vi "sv_Uniquify Collection Name.vi"(0 "tdms file ref":refnum<k34>, 5 "collection name":string="FrequencyResponse", 7 "component names":string[](array[string])=["Magnitude", "Phase", "Coherence"], 11 "error in":errorcluster, 12 "separator":string="_") -> (4 "tdms file out":refnum<k34>, 6 "unique collection name":string, 8 "unique group names (collection_component)":string[](array[string]), 15 "error out":errorcluster)   [LabVIEW 2017]
uses:
  <vilib>/addons/_NISVFA/_Shared subVIs/Controls/NI Channel Properties.ctl
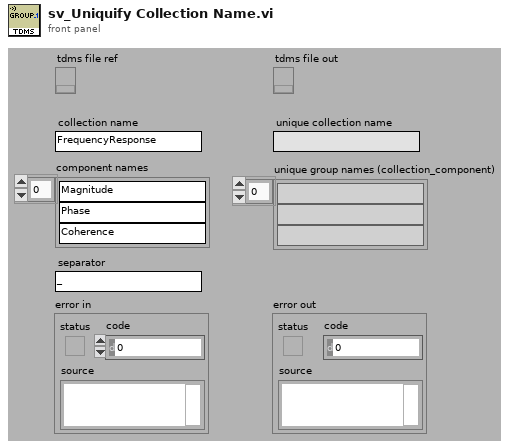
[diagram p1: front panel]
types:
  T1 = typedef "NI Channel Properties.ctl" = u16
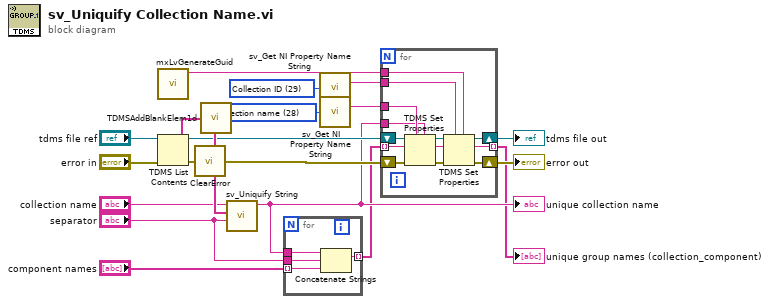
[diagram p0: block diagram]
diagram:
  w7 = T1 29 items=["Channel name", "Channel description", "Axis label", "Unit string", "Waveform X-axis label", "Waveform X-axis unit string", "x0", "dx", "Number of samples", "X channel", "Filter settled", "dB reference", "Window", "Window parameter", "Window size", "FFT size", "Peak units", "Spectrum type", "Magnitude scale", "Spectral density", "Sensor sensitivity (mV/EU)", "X-axis dimension", "LabVIEW datatype", "Function type", "Function subtype", "X values", "Independent channel", "Column index", "Collection name", "Collection ID"] ("property")
  w10 = T1 28 items=["Channel name", "Channel description", "Axis label", "Unit string", "Waveform X-axis label", "Waveform X-axis unit string", "x0", "dx", "Number of samples", "X channel", "Filter settled", "dB reference", "Window", "Window parameter", "Window size", "FFT size", "Peak units", "Spectrum type", "Magnitude scale", "Spectral density", "Sensor sensitivity (mV/EU)", "X-axis dimension", "LabVIEW datatype", "Function type", "Function subtype", "X values", "Independent channel", "Column index", "Collection name", "Collection ID"] ("property")
  n1 = call <resource>:"mxLvGenerateGuid.vi"() -> ("Value"=w2:string)  [unwired: 10 in, 1 out]
  n2 = TDMS List Contents(4:"error in", 7:"tdms file ref") -> (0:w1:errorcluster, 2:w3:string[], 3:w13:refnum<k34>)  [unwired: 1 in, 1 out]
  n3 = call <vilib>:"ClearError.vi"("error in (no error)"=w1) -> ("error out"=w14:errorcluster)
  n4 = call <vilib>:"TDMSAddBlankElem1d.vi"("input string array"=w3) -> ("output string array with blank element at the beginning"=w20:string[])
  n5 = call <vilib>:"sv_Uniquify String.vi"("separator"="separator", "reserved strings"=w20, "string"="collection name") -> ("unique string"=w8:string)  [unwired: 6 in, 2 out]
  "unique collection name" <- w8
  n6 = for {
    tunnel: "component names" -> [w22] mode=indexing
    tunnel: w8 -> [w24]
    tunnel: [w23] -> w5 mode=indexing
    tunnel: "separator" -> [w21]
    n7 = Concatenate Strings(w24, w21, w22) -> (w23:string)
  }
  n8 = call <vilib>:"sv_Get NI Property Name String.vi"("property"=w7) -> ("TDMS property name"=w6:string)  [unwired: 13 in, 1 out]
  n9 = call <vilib>:"sv_Get NI Property Name String.vi"("property"=w10) -> ("TDMS property name"=w9:string)  [unwired: 13 in, 1 out]
  n10 = for {
    tunnel: w5 -> [w30] mode=indexing
    shift-right: [w32] -> w12
    shift-left: w13 -> [w33]
    shift-right: [w31] -> w11
    shift-left: w14 -> [w34]
    tunnel: w9 -> [w29]
    tunnel: w8 -> [w28]
    tunnel: w6 -> [w27]
    tunnel: w2 -> [w26]
    tunnel: [w25] -> w4 mode=indexing
    n11 = TDMS Set Properties(5:w28, 7:w29, 8:w34, 10:w30, 11:w33) -> (0:w37:errorcluster, 2:w36:string, 3:w35:refnum<k34>)  [unwired: 1 in, 1 out]
    n12 = TDMS Set Properties(5:w26, 7:w27, 8:w37, 10:w36, 11:w35) -> (0:w31:errorcluster, 2:w25:string, 3:w32:refnum<k34>)  [unwired: 1 in, 1 out]
  }
  "tdms file out" <- w12
  "error out" <- w11
  "unique group names (collection_component)" <- w4
